vi "get channel handle - by bus channel index.vi"(7 "device type":T1=enum."LAN", 8 "error in (no error)":errorcluster, 11 "channel index(0)":u8) -> (0 "error out":errorcluster, 3 "channel handle":u16 format="%x")   [LabVIEW 2024, in "atsj peakcan basic.lvlib"]
doc: "Gets a bus channel handle for a given <b>device type </b>'s <b>channel index</b>."
uses:
  atsj peakcan basic.lvlib
  device type.ctl
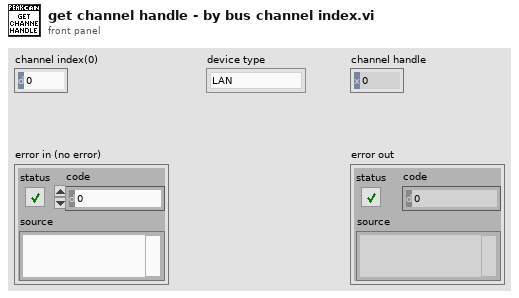
[diagram p1: front panel]
types:
  T1 = typedef "atsj peakcan basic.lvlib/device type.ctl" = enum8{"ISA", "DNG", "PCI", "USB", "PCC", "LAN"}
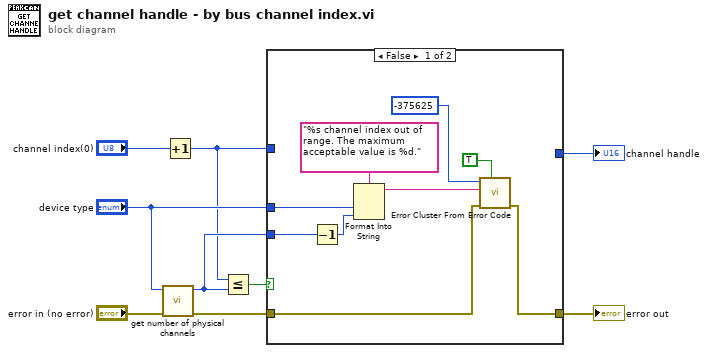
[diagram p0: block diagram]
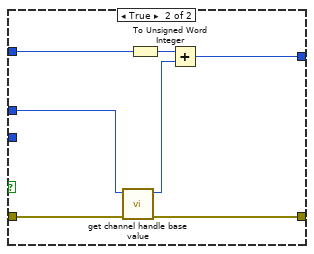
[diagram p2: hidden frame]
diagram:
  n1 = call "get number of physical channels.vi"("error in (no error)"="error in (no error)", "device type"="device type") -> ("error out"=w5:errorcluster, "number of physical channels"=w3:u8)  [unwired: 8 in]
  n2 = Increment(x="channel index(0)") -> (x+1=w1:u8)
  n3 = Less Or Equal?(x=w1, y=w3) -> (x <= y?=w2:bool)
  n4 = case shown="False" w2 {
    tunnel: w5 -> [w16 w21]
    tunnel: [w15 w22] -> w9
    tunnel: w1 -> [_ w25]
    tunnel: [_ w23] -> w8
    tunnel: w3 -> [w11 _]
    tunnel: "device type" -> [w12 w19]
    frame False {
      n5 = Decrement(x=w11) -> (x-1=w10:u8)
      n6 = Format Into String(format string="%s channel index out of range. The maximum acceptable value is %d.", w12, w10) -> (resulting string=w13:string)  [unwired: 2 in, 1 out]
      n7 = call <vilib>:"Error Cluster From Error Code.vi"("show call chain? (False)"=TRUE, "error in (no error)"=w16, "error message (\"\")"=w13, "error code (0)"=-375625) -> ("error out"=w15:errorcluster)  [unwired: 5 in]
    }
    frame True {
      n8 = call "get channel handle base value.vi"("error in (no error)"=w21, "device type"=w19) -> ("error out"=w22:errorcluster, "channel handle base value"=w20:u16)  [unwired: 8 in]
      n9 = To Unsigned Word Integer(number=w25) -> (unsigned 16bit integer=w24:u16)
      n10 = Add(x=w24, y=w20) -> (x+y=w23:u16)
    }
  }
  "error out" <- w9
  "channel handle" <- w8
